vi "Change Mouse Cursor.vi"(8 "error in (no error)":errorcluster, 10 "icon":u16(ring), 11 "VI reference (current VI)":refnum<vi>) -> (0 "error out":errorcluster)   [LabVIEW 2021]
uses:
  <vilib>/Utility/cursorutil.llb/Set Cursor (Icon Pict).vi
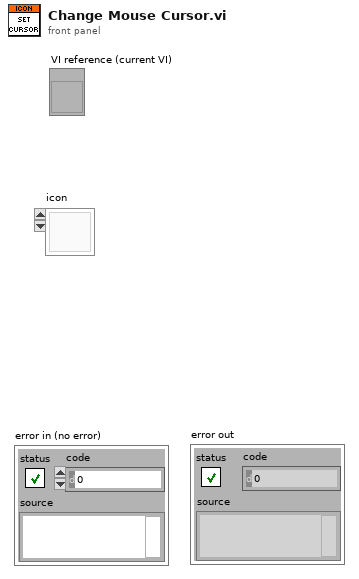
[diagram p1: front panel]
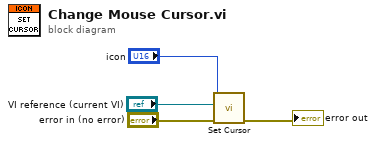
[diagram p0: block diagram]
diagram:
  n1 = call-poly <vilib>:"Set Cursor.vi"("error in (no error)"="error in (no error)", "VI reference (current VI)"="VI reference (current VI)", "icon"="icon") -> ("error out"=→"error out":errorcluster)  [unwired: 8 out]
